vi "Error 5100 - Command not found in list of commands--const.vi"() -> (0 "error out":errorcluster)   [LabVIEW 2017, in "Communications Library.lvlib"]
doc: "Error 5100\n\nError generating command to send to the DTACQ device. The array index was out of bounds; the value of the enumerated control did not match any command in \"command array--const\"."
uses:
  Communications Library.lvlib
  <vilib>/Utility/error.llb/Error Cluster From Error Code.vi
  <vilib>/ErrorRing/Error Ring.xnode
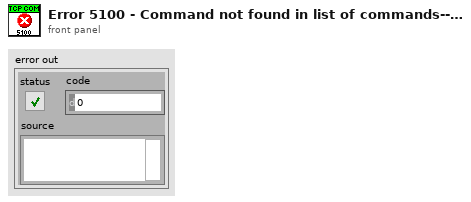
[diagram p1: front panel]
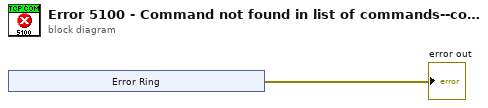
[diagram p0: block diagram]
diagram:
  n1 = xnode "Error Ring"() -> ("error out"=→"error out":errorcluster)
